vi "Saturation Mobility-Vt Calculator.vi"(9 "NumPts":dbl=5.0, 10 "Sat Id Column":dbl[](array[numeric]), 11 "Vg Column":dbl[](array[numeric])) -> (1 "XY Graph-Sat":cluster{dbl[], dbl[]}[](graph))   [LabVIEW 2011]
uses:
  <vilib>/Analysis/NI_AALPro.lvlib
panel:
  out "Width":dbl
  out "Length":dbl
  out "Capacitance (C)":dbl
  out "Index-Sat":dbl
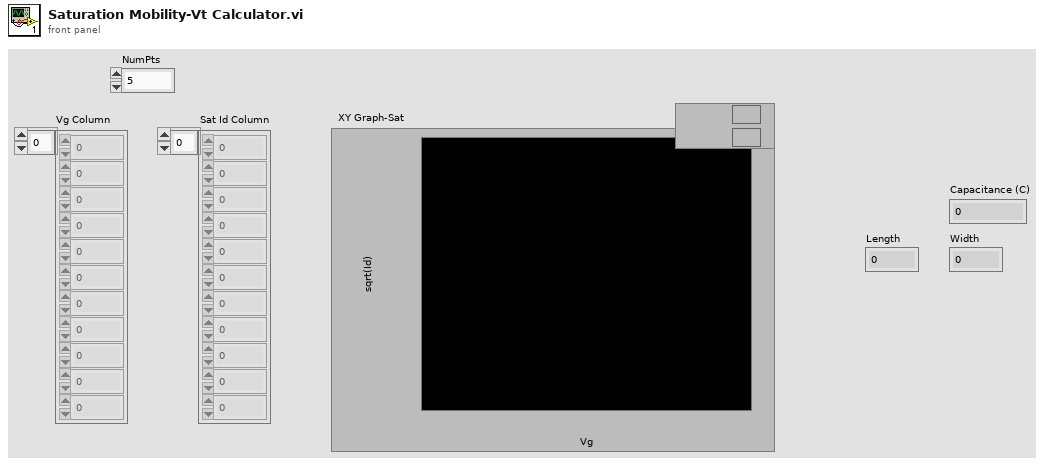
[diagram p1: front panel]
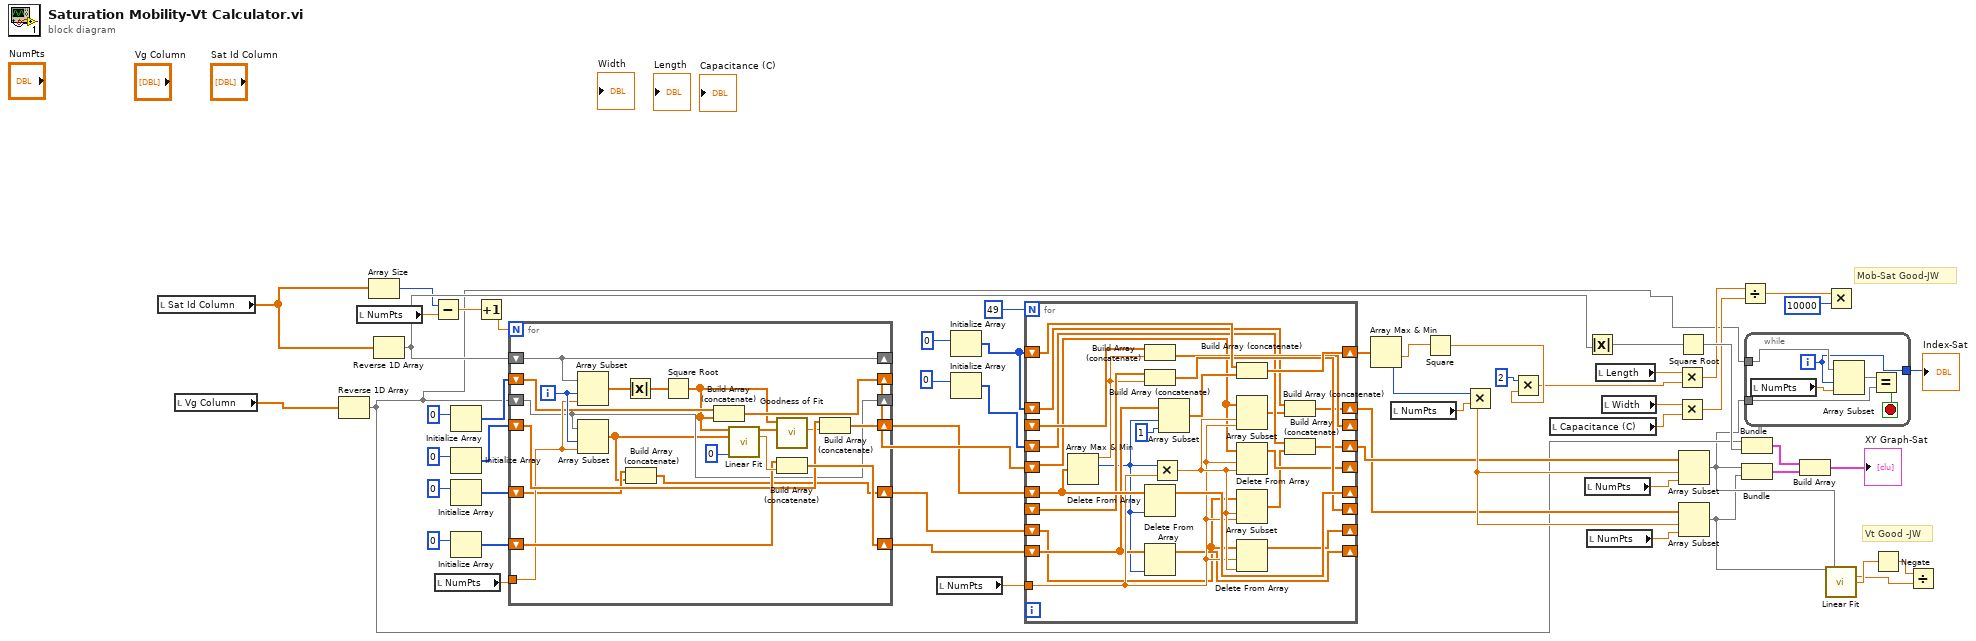
[diagram p0: block diagram]
diagram:
  # "Mob-Sat Good-JW"
  # "Vt Good -JW"
  n1 = local read "Sat Id Column"() -> (w2:dbl[])
  n2 = local read "Vg Column"() -> (w57:dbl[])
  n3 = Reverse 1D Array(array=w57) -> (reversed array=w12:dbl[])
  n4 = local read "NumPts"() -> (w51:dbl)
  n5 = Array Size(array=w2) -> (size(s)=w1:i32)
  n6 = Reverse 1D Array(array=w2) -> (reversed array=w37:dbl[])
  n7 = Subtract(x=w1, y=w51) -> (x-y=w47:dbl)
  n8 = local read "NumPts"() -> (w54:dbl)
  n9 = Initialize Array(0) -> (w33:i32[])  [unwired: 1 in]
  n10 = Initialize Array(0) -> (w21:i32[])  [unwired: 1 in]
  n11 = Initialize Array(0) -> (w34:i32[])  [unwired: 1 in]
  n12 = Initialize Array(0) -> (w20:i32[])  [unwired: 1 in]
  n13 = Increment(x=w47) -> (x+1=w48:dbl)
  n14 = for {
    N: w48 -> [_]
    shift-right: [w62] -> _
    shift-left: w12 -> [w62]
    shift-right: [w71] -> _
    shift-left: w37 -> [w71]
    shift-right: [w75] -> w26
    shift-left: w20 -> [w74]
    shift-right: [w73] -> w28
    shift-left: w21 -> [w72]
    tunnel: w54 -> [w67]
    shift-right: [w65] -> w35
    shift-left: w33 -> [w66]
    shift-right: [w63] -> w36
    shift-left: w34 -> [w64]
    i -> [w77]
    n15 = Array Subset(array=w71, index=w77, length=w67) -> (w70:dbl[])
    n16 = Array Subset(array=w62, index=w77, length=w67) -> (w61:dbl[])
    n17 = Absolute Value(x=w70) -> (abs(x)=w69:dbl[])
    n18 = Build Array (concatenate)(w64, w61) -> (w63:dbl[])
    n19 = Square Root(x=w69) -> (sqrt(x)=w58:dbl[])
    n20 = Build Array (concatenate)(w66, w58) -> (w65:dbl[])
    n21 = call <vilib>:"Linear Fit.vi"("Y"=w58, "X"=w61, "method"=0) -> ("Best Linear Fit"=w60:dbl[], "slope"=w76:dbl)  [unwired: 8 in, 3 out]
    n22 = call <vilib>:"Goodness of Fit.vi"("Best Fit"=w60, "Y"=w58) -> ("R-square"=w59:dbl)  [unwired: 6 in, 3 out]
    n23 = Build Array (concatenate)(w74, w76) -> (w75:dbl[])
    n24 = Build Array (concatenate)(w72, w59) -> (w73:dbl[])
  }
  n25 = local read "NumPts"() -> (w50:dbl)
  n26 = Initialize Array(0) -> (w43:i32[])  [unwired: 1 in]
  n27 = Initialize Array(0) -> (w38:i32[])  [unwired: 1 in]
  n28 = for {
    N: 49 -> [_]
    shift-right: [w102] -> _
    shift-left: w28 -> [w103]
    shift-right: [w82] -> _
    shift-left: w26 -> [w83]
    shift-right: [w99] -> w27
    shift-left: w43 -> [w98]
    shift-right: [w97] -> _
    shift-left: _ -> [w96]
    shift-right: [w95] -> _
    shift-left: _ -> [w94]
    shift-right: [w93] -> _
    shift-left: w35 -> [w79]
    shift-right: [w91] -> _
    shift-left: w36 -> [w78]
    tunnel: w50 -> [w90]
    shift-right: [w89] -> w40
    shift-left: w43 -> [w88]
    shift-right: [w87] -> w41
    shift-left: w38 -> [w86]
    n29 = Array Max & Min(array=w103) -> (max value=w81:dbl, max index (indices)=w80:i32)  [unwired: 2 out]
    n30 = Build Array (concatenate)(w94, w81) -> (w95:dbl[])
    n31 = Build Array (concatenate)(w96, w81) -> (w97:dbl[])
    n32 = Delete From Array(array=w103, index=w80) -> (array with subset deleted=w102:dbl[])  [unwired: 1 in, 1 out]
    n33 = Delete From Array(array=w83, index=w80) -> (array with subset deleted=w82:dbl[])  [unwired: 1 in, 1 out]
    n34 = Multiply(x=w80, y=w90) -> (x*y=w92:dbl)
    n35 = Array Subset(array=w83, index=w80, length=1) -> (w100:dbl[])
    n36 = Build Array (concatenate)(w98, w100) -> (w99:dbl[])
    n37 = Array Subset(array=w79, index=w92, length=w90) -> (w84:dbl[])
    n38 = Delete From Array(array=w79, length=w90, index=w92) -> (array with subset deleted=w93:dbl[])  [unwired: 1 out]
    n39 = Array Subset(array=w78, index=w92, length=w90) -> (w85:dbl[])
    n40 = Delete From Array(array=w78, length=w90, index=w92) -> (array with subset deleted=w91:dbl[])  [unwired: 1 out]
    n41 = Build Array (concatenate)(w88, w84) -> (w89:dbl[])
    n42 = Build Array (concatenate)(w86, w85) -> (w87:dbl[])
  }
  n43 = Array Max & Min(array=w27) -> (min value=w24:dbl, min index (indices)=w42:i32)  [unwired: 2 out]
  n44 = local read "NumPts"() -> (w53:dbl)
  n45 = Square(x=w24) -> (x^2=w19:dbl)
  n46 = Multiply(x=w42, y=w53) -> (x*y=w44:dbl)
  n47 = Multiply(x=2, y=w19) -> (x*y=w18:dbl)
  n48 = local read "Capacitance (C)"() -> (w49:dbl)
  n49 = local read "NumPts"() -> (w52:dbl)
  n50 = Absolute Value(x=w37) -> (abs(x)=w31:dbl[])
  n51 = local read "NumPts"() -> (w55:dbl)
  n52 = local read "Length"() -> (w3:dbl)
  n53 = local read "Width"() -> (w4:dbl)
  n54 = Multiply(x=w3, y=w18) -> (x*y=w17:dbl)
  n55 = Multiply(x=w4, y=w49) -> (x*y=w16:dbl)
  n56 = Square Root(x=w31) -> (sqrt(x)=w46:dbl[])
  n57 = Array Subset(array=w41, index=w44, length=w52) -> (w10:dbl[])
  n58 = Array Subset(array=w40, index=w44, length=w55) -> (w9:dbl[])
  n59 = Divide(x=w17, y=w16) -> (x/y=w14:dbl)
  n60 = Bundle(w12, w46) -> (w30:cluster{dbl[], dbl[]})  [unwired: 1 in]
  n61 = Bundle(w10, w9) -> (w45:cluster{dbl[], dbl[]})  [unwired: 1 in]
  n62 = while {
    tunnel: w12 -> [w108]
    tunnel: w10 -> [w107]
    tunnel: [w104] -> w11
    i -> [w104]
    stop <- w109 stop-if-true
    n63 = local read "NumPts"() -> (w105:dbl)
    n64 = Array Subset(array=w108, index=w104, length=w105) -> (w106:dbl[])
    n65 = Equal?(x=w106, y=w107) -> (x = y?=w109:bool)
  }
  "Index-Sat" <- w11
  n66 = Build Array(w30, w45) -> (→"XY Graph-Sat":cluster{dbl[], dbl[]}[])
  n67 = Multiply(x=w14, y=10000) -> ()  [unwired: 1 out]
  n68 = call <vilib>:"Linear Fit.vi"("Y"=w9, "X"=w10) -> ("slope"=w6:dbl, "intercept"=w8:dbl)  [unwired: 9 in, 3 out]
  n69 = Negate(x=w8) -> (-x=w7:dbl)
  n70 = Divide(x=w7, y=w6) -> ()  [unwired: 1 out]
